vi "Database Command Get Parameter Value.vi"(8 "error in (no error)":errorcluster caption="错误输入（无错误）", 10 "Index":i32, 11 "Database Command 输入":refnum<class "Database Command.lvclass"> caption="DNL_LabVIEW Object in") -> (0 "error out":errorcluster caption="错误输出", 2 "Value":variant, 3 "Database Command 输出":refnum<class "Database Command.lvclass"> caption="DNL_LabVIEW Object out")   [LabVIEW 2011, in "Database Command.lvclass"]
uses:
  Database Command.lvclass
  Database Command.lvclass/Database Command.ctl
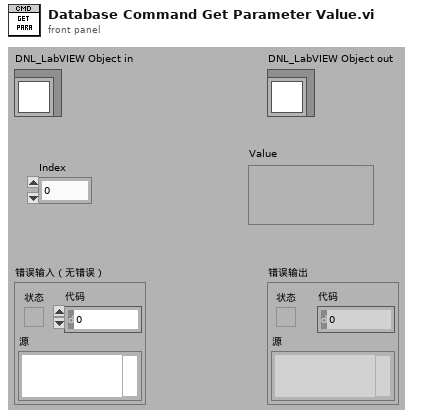
[diagram p1: front panel]
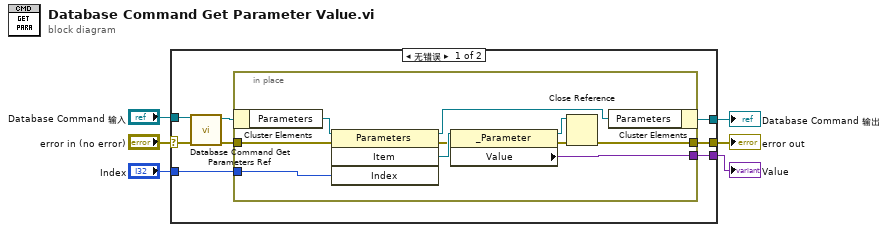
[diagram p0: block diagram]
diagram:
  n1 = case shown="无错误" "error in (no error)" {
    selector: "error in (no error)" -> [w13 w26]
    tunnel: [w7 w26] -> w5
    tunnel: [w9 w25] -> w3
    tunnel: "Database Command 输入" -> [w14 w25]
    tunnel: "Index" -> [w11 _]
    tunnel: [w10 _] -> w1
    frame No Error {
      n2 = call "Database Command Get Parameters Ref.vi"("error in (no error)"=w13, "Database Command 输入"=w14) -> ("error out"=w8:errorcluster, "Database Command 输出"=w12:refnum<class "Database Command.lvclass">)  [unwired: 8 in]
      n3 = in-place {
        in-place-border: w11 -> [w22]
        in-place-border: [w20] -> w10
        in-place-border: w8 -> [w19]
        in-place-border: [w16] -> w7
        n4 = in-place-cluster #1(w12) -> ("Parameters"=w24:refnum<k7>)
        n5 = invoke class="Parameters" method="Item"(reference=w24, error in=w19, "Index"=w22) -> (reference out=w23:refnum<k7>, error out=w18:errorcluster, "Item"=w21:refnum<k7>)  [unwired: 1 in, 1 out]
        n6 = property class="_Parameter"(reference=w21, error in=w18) -> (reference out=w15:refnum<k7>, error out=w17:errorcluster, "Value"=w20:variant)
        n7 = Close Reference(reference=w15, error in (no error)=w17) -> (error out=w16:errorcluster)
        n8 = in-place-cluster #1("Parameters"=w23) -> (w9:refnum<class "Database Command.lvclass">)
      }
    }
    frame Error {
    }
  }
  "error out" <- w5
  "Database Command 输出" <- w3
  "Value" <- w1
